vi "Do Remove From Selection.vi"(8 "error in (no error)":errorcluster, 10 "remove_from_selection Argument":T2, 11 "Data Cluster in":T1) -> (0 "error out":errorcluster, 3 "Data Cluster out":T1)   [LabVIEW 2025, in "Scripting Server.lvlib"]
uses:
  Scripting Server.lvlib
  <vilib>/ErrorRing/Error Ring.xnode
  <vilib>/Utility/error.llb/Error Cluster From Error Code.vi
  Module Data--cluster.ctl
  remove_from_selection (Reply Payload)--cluster.ctl
  remove_from_selection Argument--cluster.ctl
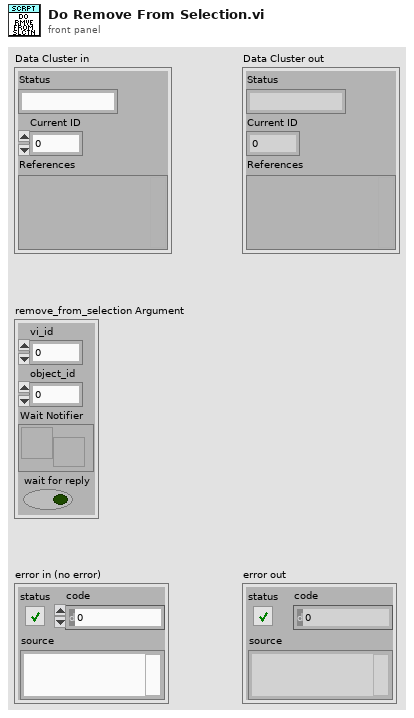
[diagram p1: front panel]
types:
  T1 = typedef "Scripting Server.lvlib/Module Data--cluster.ctl" = cluster{"Status":string, "Current ID":i32, "References":variant}
  T2 = typedef "Scripting Server.lvlib/remove_from_selection Argument--cluster.ctl" = cluster{"vi_id":i32, "object_id":i32, "Wait Notifier":refnum<notifier>, "wait for reply":bool}
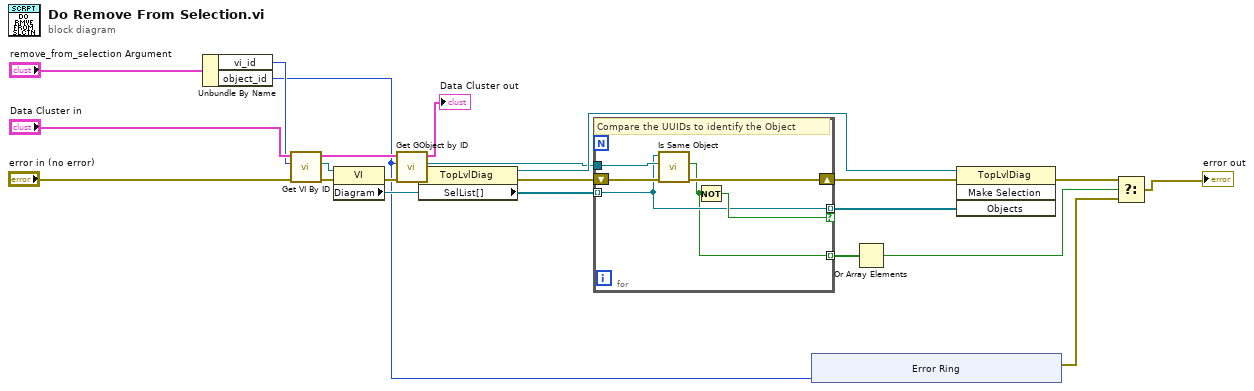
[diagram p0: block diagram]
diagram:
  n1 = Unbundle By Name("remove_from_selection Argument") -> ("vi_id"=w16:i32, "object_id"=w1:i32)
  n2 = call "Get VI By ID.vi"("error in (no error)"="error in (no error)", "ID"=w16, "Data Cluster in"="Data Cluster in") -> ("error out"=w21:errorcluster, "VI Reference"=w14:refnum<vi>, "Data Cluster out"=w18:T1)  [unwired: 6 in]
  n3 = property class="VI"(reference=w14, error in=w21) -> (error out=w15:errorcluster, "Diagram"=w12:refnum<vi>)  [unwired: 1 out]
  n4 = call "Get GObject by ID.vi"("error in (no error)"=w15, "ID"=w1, "Data Cluster in"=w18) -> ("error out"=w19:errorcluster, "gobject"=w6:refnum<vi>, "Data Cluster out"=→"Data Cluster out":T1)  [unwired: 6 in]
  n5 = property class="TopLvlDiag"(reference=w12, error in=w19) -> (reference out=w11:refnum<vi>, error out=w8:errorcluster, "SelList[]"=w10:refnum<vi>[])
  n6 = for {
    shift-right: [w29] -> w7
    shift-left: w8 -> [w28]
    tunnel: w10 -> [w25] mode=indexing
    tunnel: [w25] -> w9 mode=indexing if=w27
    tunnel: w6 -> [w26]
    tunnel: [w24] -> w3 mode=indexing
    # "Compare the UUIDs to identify the Object"
    n7 = call "Is Same Object.vi"("error in (no error)"=w28, "values"=w26, "GObject in"=w25) -> ("error out"=w29:errorcluster, "Same"=w24:bool)  [unwired: 7 in]
    n8 = Not(x=w24) -> (.not. x?=w27:bool)
  }
  n9 = xnode "Error Ring"("parameter 0"=w1) -> ("error out"=w4:errorcluster)
  n10 = Or Array Elements(Boolean array=w3) -> (logical OR=w2:bool)
  n11 = invoke class="TopLvlDiag" method="Make Selection"(reference=w11, error in=w7, "Objects"=w9) -> (error out=w13:errorcluster)  [unwired: 1 in, 3 out]
  n12 = Select(t=w13, s=w2, f=w4) -> (s? t:f=→"error out":errorcluster)
